vi "sin.vi"() -> ()   [LabVIEW 2014]
uses:
  <vilib>/measure/NI_MABase.lvlib
panel:
  out "Waveform Graph":waveform(dbl)(graph)
  in  "freq":dbl format="%#_13g"
  in  "amp":dbl format="%#_13g"
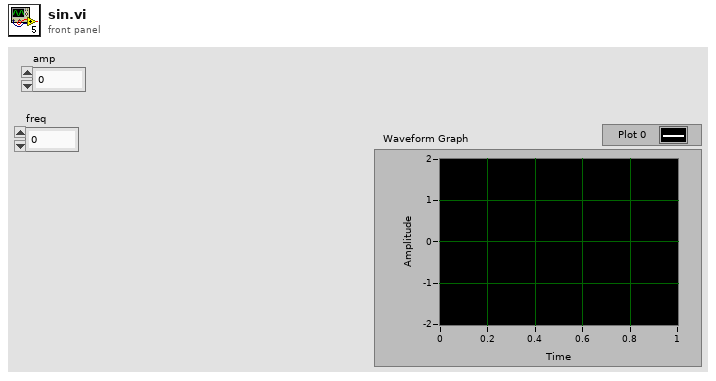
[diagram p1: front panel]
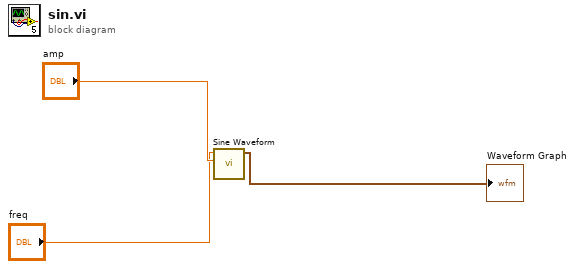
[diagram p0: block diagram]
diagram:
  n1 = call <vilib>:"Sine Waveform.vi"("amplitude"="amp", "frequency"="freq") -> ("signal out"=→"Waveform Graph":waveform(dbl))  [unwired: 8 in, 1 out]
